vi "CheckUnbefitting__slk_mt.vi"(8 "error in (no error)":errorcluster, 11 "label in":refnum<class "Label__slk_mt.lvclass">) -> (0 "error out":errorcluster, 2 "unbefitting?":bool, 3 "label out":refnum<class "Label__slk_mt.lvclass">)   [LabVIEW 2020, in "Label__slk_mt.lvclass"]
doc: "Checks if the label is unbefitting."
uses:
  Label__slk_mt.lvclass
  Label__slk_mt.lvclass/Label__slk_mt.ctl
  Segment/Segment__slk_mt.lvclass
panel:
  # "CheckUnbefitting__slk_mt.vi\nChecks if the label is unbefitting.\n\nNOTICE -- YOU MUST LEAVE THIS NOTICE IN PLACE.\n\nCopyright (c) 2011, LIANG LIU Shawn.Liu.cn@gmail.com\nAll rights reserved.\n\nRedistribution and use in source and binary forms, with or without modification, are permitted provided that the following conditions are met:\n-Redistributions of source code must retain the above copyright notice, this list of conditions and the following disclaimer.\n-Redistributions in binary form must reproduce the above copyright notice, this list of conditions and the following disclaimer in the documentation and/or other materials provided with the distribution.\n-Neither the name of the eLp nor the names of its contributors may be used to endorse or promote products derived from this software without specific prior written permission.\n\nTHIS SOFTWARE IS PROVIDED BY THE COPYRIGHT HOLDERS AND CONTRIBUTORS \"AS IS\" AND ANY EXPRESS OR IMPLIED WARRANTIES, INCLUDING, BUT NOT LIMITED TO, THE IMPLIED WARRANTIES OF MERCHANTABILITY AND FITNESS FOR A PARTICULAR PURPOSE ARE DISCLAIMED. IN NO EVENT SHALL THE COPYRIGHT HOLDER OR CONTRIBUTORS BE LIABLE FOR ANY DIRECT, INDIRECT, INCIDENTAL, SPECIAL, EXEMPLARY, OR CONSEQUENTIAL DAMAGES (INCLUDING, BUT NOT LIMITED TO, PROCUREMENT OF SUBSTITUTE GOODS OR SERVICES; LOSS OF USE, DATA, OR PROFITS; OR BUSINESS INTERRUPTION) HOWEVER CAUSED AND ON ANY THEORY OF LIABILITY, WHETHER IN CONTRACT, STRICT LIABILITY, OR TORT (INCLUDING NEGLIGENCE OR OTHERWISE) ARISING IN ANY WAY OUT OF THE USE OF THIS SOFTWARE, EVEN IF ADVISED OF THE POSSIBILITY OF SUCH DAMAGE."
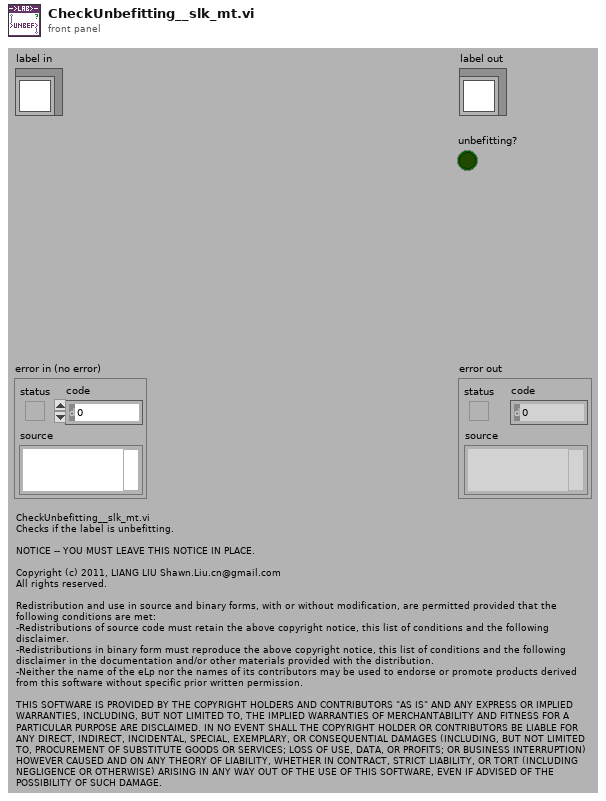
[diagram p1: front panel]
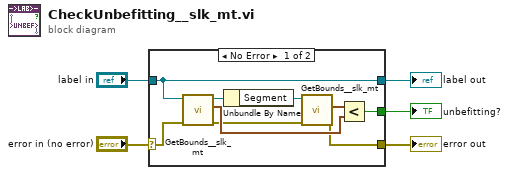
[diagram p0: block diagram]
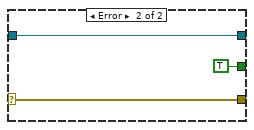
[diagram p2: hidden frame]
diagram:
  n1 = case shown="No Error" "error in (no error)" {
    selector: "error in (no error)" -> [w8 w17]
    tunnel: [w6 w17] -> w4
    tunnel: [w11 w16] -> w2
    tunnel: "label in" -> [w11 w16]
    tunnel: [w7 TRUE] -> w1
    frame No Error {
      n2 = call "GetBounds__slk_mt.vi"("error in (no error)"=w8, "label in"=w11) -> ("error out"=w12:errorcluster, "bounds"=w13:cluster{"Width":u32, "Height":u32}, "label out"=w10:refnum<class "Label__slk_mt.lvclass">)  [unwired: 7 in]
      n3 = Unbundle By Name(w10) -> ("Segment"=w9:refnum<class "Segment__slk_mt.lvclass">)
      n4 = call "GetBounds__slk_mt.vi"("error in (no error)"=w12, "segment in"=w9) -> ("error out"=w6:errorcluster, "bounds"=w14:cluster{"Width":u32, "Height":u32})  [unwired: 7 in, 1 out]
      n5 = Less?(x=w14, y=w13) -> (x < y?=w7:bool)
    }
    frame Error {
    }
  }
  "error out" <- w4
  "label out" <- w2
  "unbefitting?" <- w1
